vi "Acquire waveform.vi"(7 "Source":T1(ring), 8 "Error In":errorcluster, 11 "VISA Resource In":refnum<visa-resource-name>) -> (0 "Error Out":errorcluster, 1 "Waveform":waveform(dbl), 3 "VISA Resource Out":refnum<visa-resource-name>)   [LabVIEW 2015]
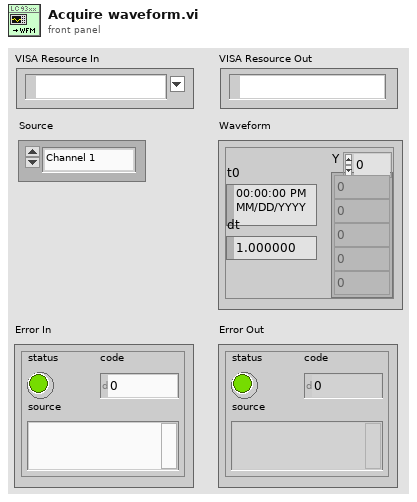
[diagram p1: front panel]
types:
  T1 = enum16{"Channel 1", "Channel 2", "Channel 3", "Channel 4", "Memory 1", "Memory 2", "Memory 3", "Memory 4", "Trace A", "Trace B", "Trace C", "Trace D"}
  T2 = cluster{"t(0) (sec)":ext, "Delta t (sec)":dbl, "Amplitude Array (Volts)":sgl[]}
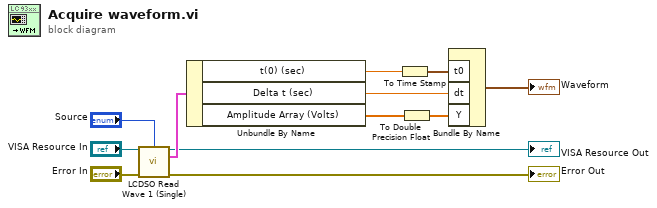
[diagram p0: block diagram]
diagram:
  n1 = call <instrlib>:"LCDSO Read Wave 1 (Single).vi"("VISA session"="VISA Resource In", "Source (0:Ch. 1)"="Source", "error in (no error)"="Error In") -> ("dup VISA session"=→"VISA Resource Out":refnum<visa-resource-name>, "Wave Output"=w9:T2, "error out"=→"Error Out":errorcluster)  [unwired: 7 in, 3 out]
  n2 = Unbundle By Name(w9) -> ("t(0) (sec)"=w11:ext, "Delta t (sec)"=w10:dbl, "Amplitude Array (Volts)"=w1:sgl[])
  n3 = To Time Stamp(1:w11) -> (0:w12:timestamp)
  n4 = To Double Precision Float(number=w1) -> (double precision float=w2:dbl[])
  n5 = Bundle By Name("t0"=w12, "dt"=w10, "Y"=w2) -> (→"Waveform":waveform(dbl))  [unwired: 1 in]
